vi "Launcher.vi"() -> ()   [LabVIEW 2012]
uses:
  StateMachineEnum.ctl
  Robot Global Data.vi
panel:
  in  "PID R":T1={"proportional gain (Kc)"=0.0008, "integral time (Ti, min)"=0.010000000000000009, "derivative time (Td, min)"=0.0} {"derivative time (Td, min)" step=0.01 format="%.2f"; "integral time (Ti, min)" step=0.01 format="%.2f"; "proportional gain (Kc)" step=0.0001 format="%.4f"}
  in  "Output R":cluster{"output high":dbl, "output low":dbl}={"output high"=1.0, "output low"=0.0} {"output low" step=0.1 format="%.2f"; "output high" step=0.1 format="%.2f"}
  in  "PID L":T1={"proportional gain (Kc)"=0.0008, "integral time (Ti, min)"=0.01, "derivative time (Td, min)"=0.0} {"derivative time (Td, min)" step=0.01 format="%.2f"; "integral time (Ti, min)" step=0.01 format="%.2f"; "proportional gain (Kc)" step=0.0001 format="%.4f"}
  in  "Output L":cluster{"output high":dbl, "output low":dbl}={"output high"=1.0, "output low"=0.0} {"output low" step=0.1 format="%.2f"; "output high" step=0.1 format="%.2f"}
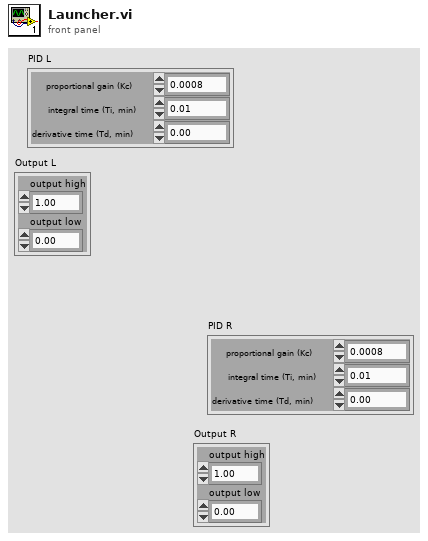
[diagram p1: front panel]
types:
  T1 = cluster{"proportional gain (Kc)":dbl, "integral time (Ti, min)":dbl, "derivative time (Td, min)":dbl}
  T2 = typedef "StateMachineEnum.ctl" = enum16{"Init", "Idle", "Start", "Do", "Stop"}
  T3 = typedef "WPI_MotorControlDeviceRef.ctl" = cluster{"DeviceStatus":errorcluster, "Type":enum16{"PWM", "CAN"}, "PWM":cluster{"Digital Module":T4, "PWM Channel":T5, "DeadBand":T6}, "CAN":cluster{"Device Number":u8, "Control Mode":T7, "Semaphore":T8, "Max Vout":dbl}, "Invert":bool, "TransformRef":T9, "InvTransformRef":T9}
  T4 = typedef "FPGA_TypedefDigitalModule.ctl" = enum16{"Digital Module 1", "Digital Module 2"}
  T5 = typedef "FPGA_DIOPWMChannel.ctl" = enum8{"PWM 1", "PWM 2", "PWM 3", "PWM 4", "PWM 5", "PWM 6", "PWM 7", "PWM 8", "PWM 9", "PWM 10", "Invalid"}
  T6 = typedef "WPI_PWMDeadband.ctl" = cluster{"Name":string, "maxPositivePwm":i32, "minPositivePwm":i32, "centerPwm":i32, "maxNegativePwm":i32, "minNegativePwm":i32, "angularRange":u16}
  T7 = typedef "WPI_CANJaguar_ControlMode.ctl" = enum8{"Percent VBus", "Current", "Speed", "Position", "Voltage"}
  T8 = typedef "Semaphore RefNum" = refnum<k1>
  T9 = typedef "WPI_PWMTransform_ConPane.ctl" = refnum<vi>
  T10 = typedef "WPI_CounterDevRef.ctl" = cluster{"DevStatus":errorcluster, "CntIndex":T11}
  T11 = typedef "FPGA_CounterCtrSystemIndex.ctl" = enum8{"Ctr 0", "Ctr 1", "Ctr 2", "Ctr 3", "Ctr 4", "Ctr 5", "Ctr 6", "Ctr 7", "Invalid"}
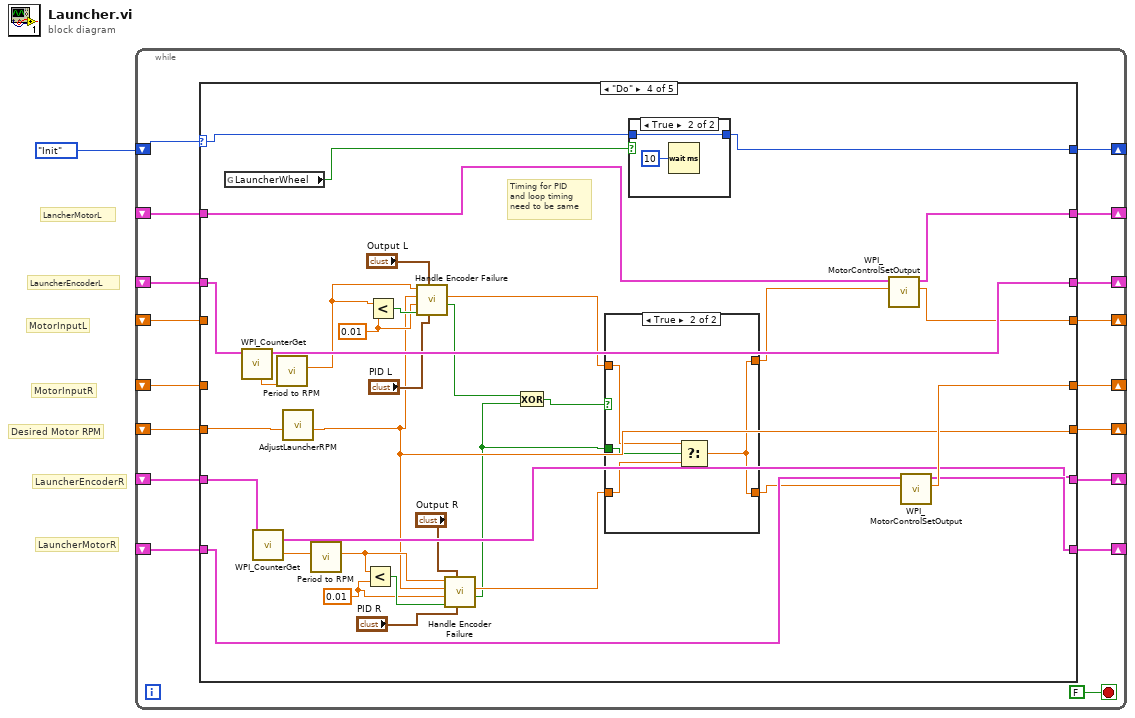
[diagram p0: block diagram]
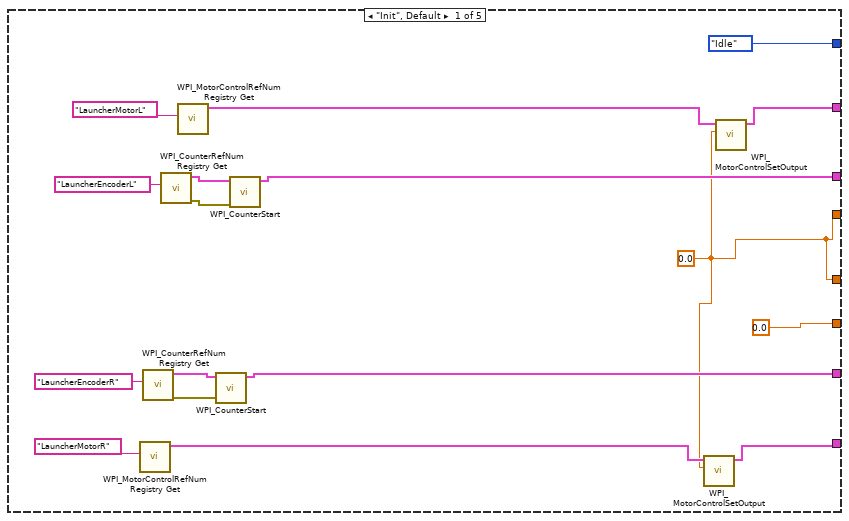
[diagram p2: hidden frame]
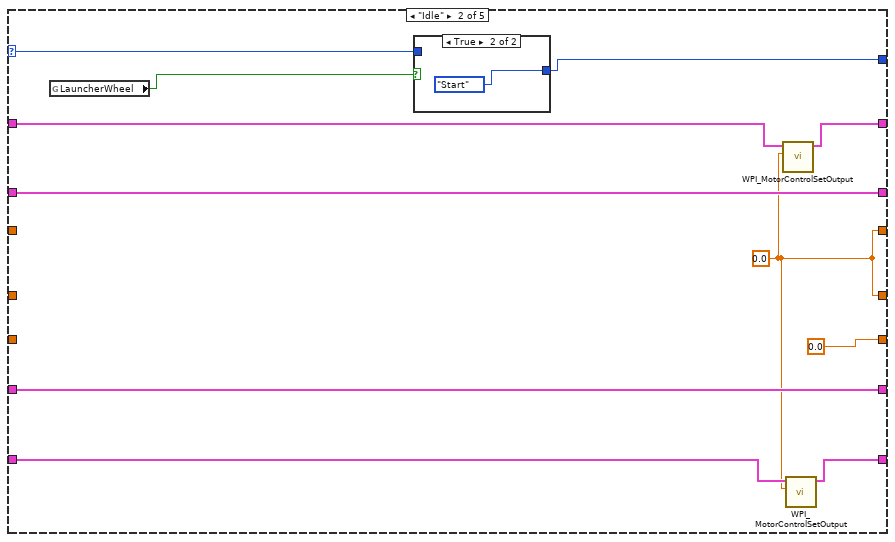
[diagram p3: hidden frame]
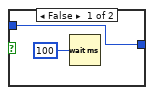
[diagram p4: hidden frame]
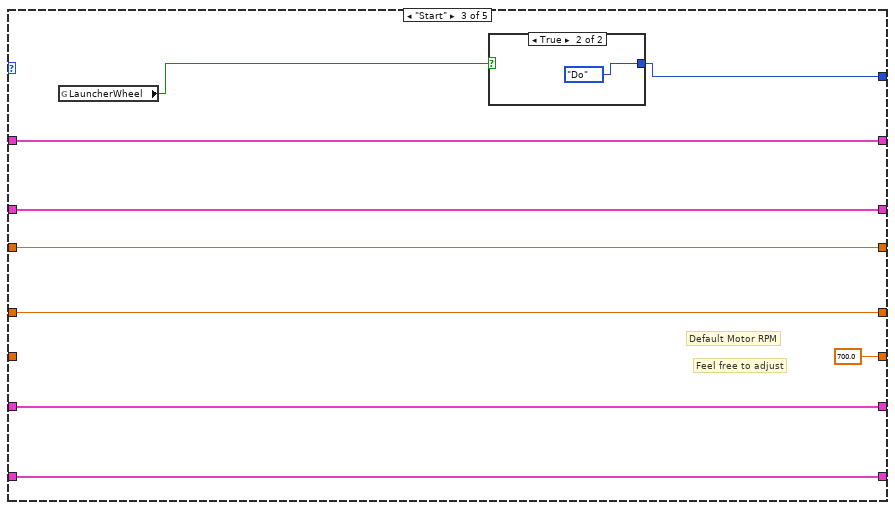
[diagram p5: hidden frame]
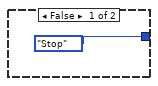
[diagram p6: hidden frame]
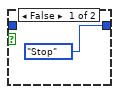
[diagram p8: hidden frame]
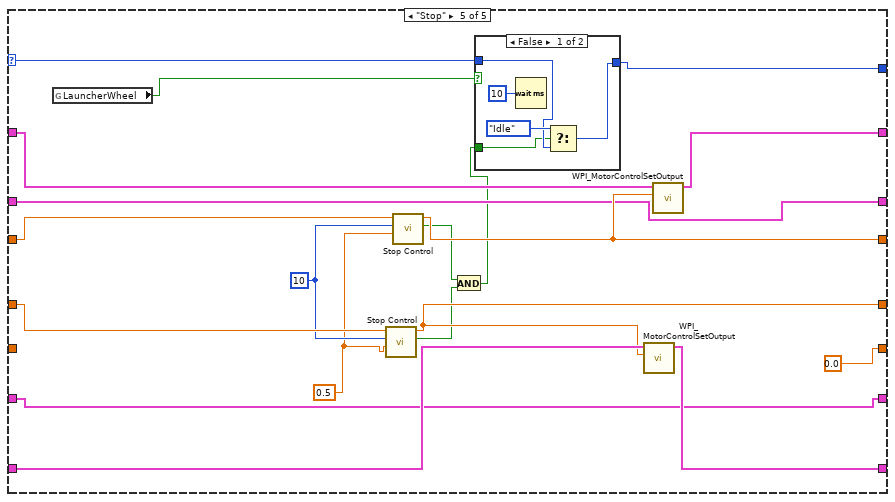
[diagram p9: hidden frame]
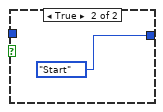
[diagram p10: hidden frame]
diagram:
  # "Desired Motor RPM"
  # "MotorInputR"
  # "MotorInputL"
  # "LauncherMotorR"
  # "LauncherEncoderR"
  # "LauncherEncoderL"
  # "LancherMotorL"
  n1 = while {
    shift-right: [w17] -> _
    shift-left: _ -> [w7]
    shift-right: [w16] -> _
    shift-left: _ -> [w8]
    shift-right: [w15] -> _
    shift-left: _ -> [w6]
    shift-right: [w14] -> _
    shift-left: _ -> [w5]
    shift-right: [w13] -> _
    shift-left: StateMachineEnum."Init" ("State") -> [w18]
    shift-right: [w12] -> _
    shift-left: _ -> [w10]
    shift-right: [w11] -> _
    shift-left: _ -> [w9]
    shift-right: [w3] -> _
    shift-left: _ -> [w2]
    stop <- FALSE stop-if-true
    n2 = case shown="\"Do\"" w18 {
      selector: w18 -> [_ w45 _ w93 w121]
      tunnel: [w23 w40 w56 w84 w114] -> w17
      tunnel: [w25 w43 w55 w81 w113] -> w16
      tunnel: [w29 w42 w54 w82 w109] -> w15
      tunnel: [w21 w38 w53 w83 w110] -> w14
      tunnel: [StateMachineEnum."Idle" ("State") w44 w57 w92 w120] -> w13
      tunnel: [w20 w37 w52 w80 w115] -> w12
      tunnel: [w20 w37 w51 w85 w111] -> w11
      tunnel: w10 -> [_ _ w52 _ w119]
      tunnel: w9 -> [_ _ w51 _ w118]
      tunnel: w8 -> [_ w43 w55 w89 w113]
      tunnel: w7 -> [_ w41 w56 w86 w116]
      tunnel: w6 -> [_ w42 w54 w88 w109]
      tunnel: w5 -> [_ w39 w53 w87 w112]
      tunnel: [0.0 ("y") 0.0 ("y") 700.0 w69 0.0 ("y")] -> w3
      tunnel: w2 -> [_ _ _ w79 _]
      frame "Init", Default {
        w20 = 0.0
        n3 = call <vilib>:"WPI_MotorControlRefNum Registry Get.vi"("refnum name"="LauncherMotorR") -> ("MotorControlDevRef"=w22:T3)  [unwired: 9 in, 1 out]
        n4 = call <vilib>:"WPI_CounterRefNum Registry Get.vi"("refnum name"="LauncherEncoderR") -> ("error out"=w28:errorcluster, "CounterDevRef"=w30:T10)  [unwired: 9 in]
        n5 = call <vilib>:"WPI_CounterRefNum Registry Get.vi"("refnum name"="LauncherEncoderL") -> ("error out"=w26:errorcluster, "CounterDevRef"=w27:T10)  [unwired: 9 in]
        n6 = call <vilib>:"WPI_MotorControlRefNum Registry Get.vi"("refnum name"="LauncherMotorL") -> ("MotorControlDevRef"=w24:T3)  [unwired: 9 in, 1 out]
        n7 = call <vilib>:"WPI_CounterStart.vi"("error in (no error)"=w28, "CounterDevRef in"=w30) -> ("CounterDevRef out"=w29:T10)  [unwired: 8 in, 1 out]
        n8 = call <vilib>:"WPI_CounterStart.vi"("error in (no error)"=w26, "CounterDevRef in"=w27) -> ("CounterDevRef out"=w25:T10)  [unwired: 8 in, 1 out]
        n9 = call <vilib>:"WPI_MotorControlSetOutput.vi"("Output"=w20, "MotorControlDevRef"=w22) -> ("MotorControlDevRef"=w21:T3)  [unwired: 7 in, 2 out]
        n10 = call <vilib>:"WPI_MotorControlSetOutput.vi"("Output"=w20, "MotorControlDevRef"=w24) -> ("MotorControlDevRef"=w23:T3)  [unwired: 7 in, 2 out]
      }
      frame "Idle" {
        w37 = 0.0
        n11 = global read "Robot Global Data.vi" "LauncherWheel"() -> (w46:bool)
        n12 = case shown="True" w46 {
          tunnel: w45 -> [w48 _]
          tunnel: [w48 StateMachineEnum."Start" ("State")] -> w44
          frame False {
            n13 = Wait (ms)(milliseconds to wait=u32 100) -> ()  [unwired: 1 out]
          }
          frame True {
          }
        }
        n14 = call <vilib>:"WPI_MotorControlSetOutput.vi"("Output"=w37, "MotorControlDevRef"=w41) -> ("MotorControlDevRef"=w40:T3)  [unwired: 7 in, 2 out]
        n15 = call <vilib>:"WPI_MotorControlSetOutput.vi"("Output"=w37, "MotorControlDevRef"=w39) -> ("MotorControlDevRef"=w38:T3)  [unwired: 7 in, 2 out]
      }
      frame "Start" {
        # "Feel free to adjust"
        # "Default Motor RPM"
        n16 = global read "Robot Global Data.vi" "LauncherWheel"() -> (w58:bool)
        n17 = case shown="True" w58 {
          tunnel: [StateMachineEnum."Stop" ("State") StateMachineEnum."Do" ("State")] -> w57
          frame False {
          }
          frame True {
          }
        }
      }
      frame "Do" {
        w70 = 0.01
        w75 = 0.01
        # "Timing for PID\nand loop timing\nneed to be same"
        n18 = global read "Robot Global Data.vi" "LauncherWheel"() -> (w94:bool)
        n19 = call <vilib>:"WPI_CounterGet.vi"("CounterDevRef in"=w89) -> ("CounterDevRef out"=w81:T10, "Period (sec)"=w90:dbl)  [unwired: 5 in, 4 out]
        n20 = call <vilib>:"WPI_CounterGet.vi"("CounterDevRef in"=w88) -> ("CounterDevRef out"=w82:T10, "Period (sec)"=w91:dbl)  [unwired: 5 in, 4 out]
        n21 = call "Period to RPM.vi"("Period (sec)"=w90) -> ("RPM"=w68:dbl)  [unwired: 10 in]
        n22 = call "AdjustLauncherRPM.vi"("Current RPM"=w79) -> ("New RPM"=w69:dbl)  [unwired: 10 in]
        n23 = call "Period to RPM.vi"("Period (sec)"=w91) -> ("RPM"=w74:dbl)  [unwired: 10 in]
        n24 = Less?(x=w74, y=w75) -> (x < y?=w76:bool)
        n25 = Less?(x=w68, y=w70) -> (x < y?=w71:bool)
        n26 = call "Handle Encoder Failure.vi"("PID gains"="PID L", "Output Range"="Output L", "Encoder Failure"=w71, "Loop Time"=w70, "Desired RPM"=w69, "Current RPM"=w68) -> ("Encoder Failure Out"=w62:bool, "Motor Output"=w66:dbl)  [unwired: 4 in]
        n27 = call "Handle Encoder Failure.vi"("PID gains"="PID R", "Output Range"="Output R", "Encoder Failure"=w76, "Loop Time"=w75, "Desired RPM"=w69, "Current RPM"=w74) -> ("Encoder Failure Out"=w61:bool, "Motor Output"=w65:dbl)  [unwired: 4 in]
        n28 = Exclusive Or(1:w61, 2:w62) -> (0:w67:bool)
        n29 = case shown="True" w67 {
          tunnel: w66 -> [w96 w98]
          tunnel: w65 -> [w95 w99]
          tunnel: [w95 w97] -> w64
          tunnel: [w96 w97] -> w63
          tunnel: w61 -> [_ w100]
          frame False {
          }
          frame True {
            n30 = Select(t=w98, s=w100, f=w99) -> (s? t:f=w97:dbl)
          }
        }
        n31 = case shown="True" w94 {
          tunnel: w93 -> [_ w102]
          tunnel: [StateMachineEnum."Stop" ("State") w102] -> w92
          frame False {
          }
          frame True {
            n32 = Wait (ms)(milliseconds to wait=u32 10) -> ()  [unwired: 1 out]
          }
        }
        n33 = call <vilib>:"WPI_MotorControlSetOutput.vi"("Output"=w63, "MotorControlDevRef"=w86) -> ("Motor Output"=w80:dbl, "MotorControlDevRef"=w84:T3)  [unwired: 7 in, 1 out]
        n34 = call <vilib>:"WPI_MotorControlSetOutput.vi"("Output"=w64, "MotorControlDevRef"=w87) -> ("Motor Output"=w85:dbl, "MotorControlDevRef"=w83:T3)  [unwired: 7 in, 1 out]
      }
      frame "Stop" {
        w105 = 0.5 ("y")
        w117 = u32 10 ("milliseconds to wait")
        n35 = global read "Robot Global Data.vi" "LauncherWheel"() -> (w122:bool)
        n36 = call "Stop Control.vi"("Rate (unit/s)"=w105, "Loop Time (ms)"=w117, "Recieved Motor Input"=w118) -> ("Done Stopping"=w107:bool, "New Motor Input"=w111:dbl)  [unwired: 7 in]
        n37 = call "Stop Control.vi"("Rate (unit/s)"=w105, "Loop Time (ms)"=w117, "Recieved Motor Input"=w119) -> ("Done Stopping"=w108:bool, "New Motor Input"=w115:dbl)  [unwired: 7 in]
        n38 = And(x=w108, y=w107) -> (x .and. y?=w106:bool)
        n39 = case shown="False" w122 {
          tunnel: w121 -> [w125 _]
          tunnel: [w124 StateMachineEnum."Start" ("State")] -> w120
          tunnel: w106 -> [w123 _]
          frame False {
            n40 = Wait (ms)(milliseconds to wait=u32 10) -> ()  [unwired: 1 out]
            n41 = Select(t=StateMachineEnum."Idle" ("State"), s=w123, f=w125) -> (s? t:f=w124:T2)
          }
          frame True {
          }
        }
        n42 = call <vilib>:"WPI_MotorControlSetOutput.vi"("Output"=w111, "MotorControlDevRef"=w112) -> ("MotorControlDevRef"=w110:T3)  [unwired: 7 in, 2 out]
        n43 = call <vilib>:"WPI_MotorControlSetOutput.vi"("Output"=w115, "MotorControlDevRef"=w116) -> ("MotorControlDevRef"=w114:T3)  [unwired: 7 in, 2 out]
      }
    }
  }
